vi "Initialize.vi"(8 "error in (no error)":errorcluster, 10 "Controller":T2) -> (0 "error out":errorcluster, 3 "Pump":T1)   [LabVIEW 2017, in "Pump Controller.lvlib"]
uses:
  Pump Controller.lvlib
  <instrlib>/Roboteq Controller KBL1xxx/Public/Controls/Controller.ctl
  Controls/Pump.ctl
  <instrlib>/Roboteq Controller KBL1xxx/Roboteq Controller KBL1xxx.lvlib
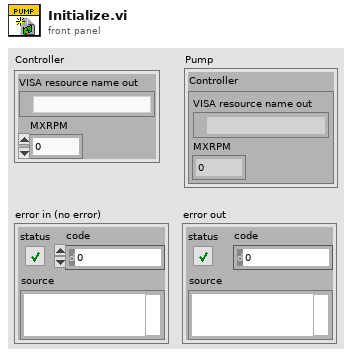
[diagram p1: front panel]
types:
  T1 = typedef "Pump Controller.lvlib/Pump.ctl" = cluster{"Controller":T2}
  T2 = typedef "Roboteq Controller KBL1xxx.lvlib/Controller.ctl" = cluster{"VISA resource name out":refnum<visa-resource-name>, "MXRPM":u16}
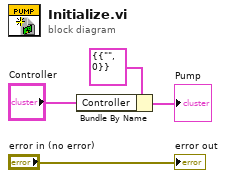
[diagram p0: block diagram]
diagram:
  n1 = Bundle By Name(cluster=T1 {"Controller"={"VISA resource name out"="", "MXRPM"=0}} ("Pump"), "Controller"="Controller") -> (→"Pump":T1)
  "error out" <- "error in (no error)"
